vi "intensity_calibration2.vi"() -> ()   [LabVIEW 2014]
uses:
  <vilib>/Utility/file.llb/Read From Spreadsheet File (DBL).vi
panel:
  in  "reference":refnum<vi>
  in  "Array":u16[][](array[numeric])
  out "min value":dbl
  out "max value":dbl
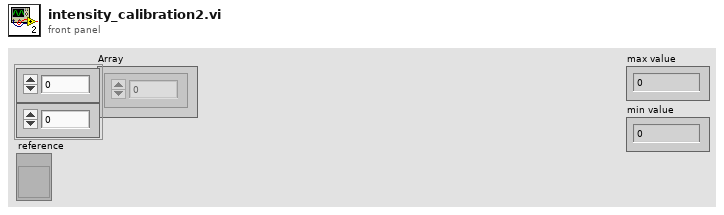
[diagram p1: front panel]
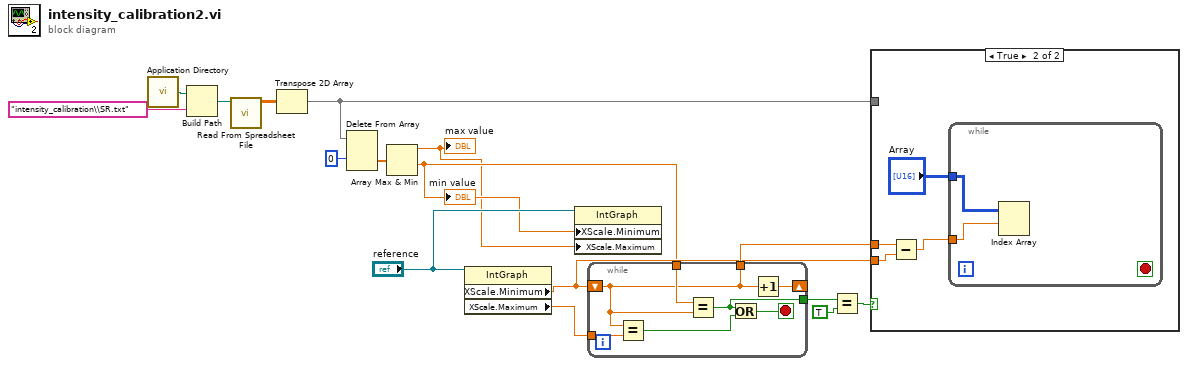
[diagram p0: block diagram]
diagram:
  n1 = call <vilib>:"Application Directory.vi"() -> ("Application Directory"=w16:path)
  n2 = Build Path(base path=w16, name or relative path="intensity_calibration\\SR.txt") -> (appended path=w15:path)
  n3 = call-poly <vilib>:"Read From Spreadsheet File.vi"("file path (dialog if empty)"=w15) -> ("all rows"=w11:dbl[][])  [unwired: 6 in, 4 out]
  n4 = Transpose 2D Array(2D array=w11) -> (transposed array=w4:dbl[][])
  n5 = Delete From Array(array=w4, index (row)=0) -> (deleted portion=w12:dbl[])  [unwired: 2 in, 1 out]
  n6 = Array Max & Min(array=w12) -> (max value=w1:dbl, min value=w2:dbl)  [unwired: 2 out]
  "max value" <- w1
  "min value" <- w2
  n7 = property on="Property Node" class="IntGraph"(reference="reference") -> ("XScale.Minimum"=w5:dbl, "XScale.Maximum"=w10:dbl)  [unwired: 1 in, 2 out]
  n8 = property on="Property Node" class="IntGraph"(reference="reference", "XScale.Minimum"=w2, "XScale.Maximum"=w1) -> ()  [unwired: 1 in, 2 out]
  n9 = while {
    tunnel: w2 -> [w23]
    tunnel: w10 -> [w21]
    shift-right: [w22] -> _
    shift-left: w5 -> [w17]
    tunnel: [w18] -> w9
    tunnel: [w17] -> w6
    stop <- w19 stop-if-true
    n10 = Equal?(x=w17, y=w21) -> (x = y?=w20:bool)
    n11 = Equal?(x=w23, y=w17) -> (x = y?=w18:bool)
    n12 = Or(x=w18, y=w20) -> (x .or. y?=w19:bool)
    n13 = Increment(x=w17) -> (x+1=w22:dbl)
  }
  n14 = Equal?(x=w9, y=TRUE) -> (x = y?=w7:bool)
  n15 = case shown="True" w7 {
    tunnel: w6 -> [_ w27]
    tunnel: w5 -> [_ w26]
    tunnel: w4 -> [_ _]
    frame False {
    }
    frame True {
      n16 = Subtract(x=w27, y=w26) -> (x-y=w24:dbl)
      n17 = while {
        tunnel: "Array" -> [w29]
        tunnel: w24 -> [w28]
        stop <- _ stop-if-true
        n18 = Index Array(array=w29, index (row)=w28) -> ()  [unwired: 1 in, 1 out]
      }
    }
  }
